vi "Write Data.vi"(8 "error in (no error)":errorcluster, 10 "Data":T1, 11 "Alicat Data in":refnum<class "Alicat Data.lvclass">) -> (0 "error out":errorcluster, 3 "Alicat Data out":refnum<class "Alicat Data.lvclass">)   [LabVIEW 2015, in "Alicat Lib.lvlib" / "Alicat Data.lvclass"]
uses:
  Alicat Data.lvclass
  Alicat Data.lvclass/Alicat Data.ctl
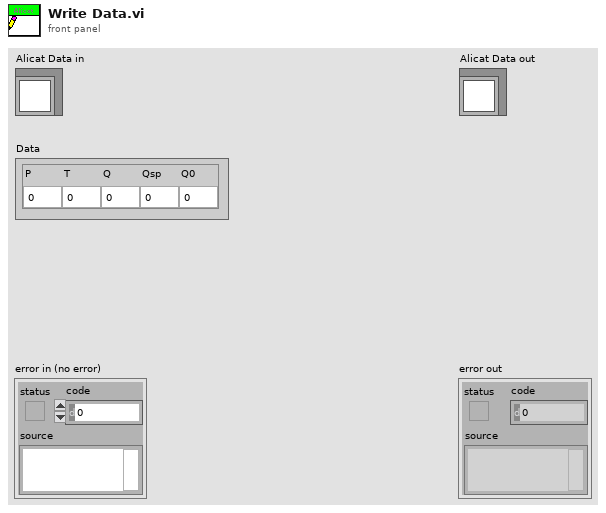
[diagram p1: front panel]
types:
  T1 = cluster{"P":sgl, "T":sgl, "Q":sgl, "Qsp":sgl, "Q0":sgl}
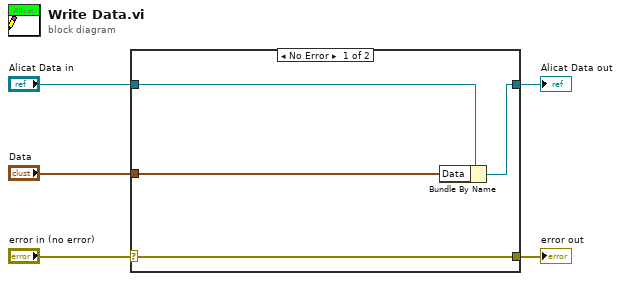
[diagram p0: block diagram]
diagram:
  n1 = case shown="No Error" "error in (no error)" {
    selector: "error in (no error)" -> [w9 w10]
    tunnel: [w9 w10] -> w4
    tunnel: [w7 w11] -> w2
    tunnel: "Alicat Data in" -> [w8 w11]
    tunnel: "Data" -> [w6 _]
    frame No Error {
      n2 = Bundle By Name(cluster=w8, "Data"=w6) -> (w7:refnum<class "Alicat Data.lvclass">)
    }
    frame Error {
    }
  }
  "error out" <- w4
  "Alicat Data out" <- w2
